vi "macro_FlyWheel_Sim_Execute.vi"() -> ()   [LabVIEW 2019, in "Trajectory_Library.lvlib"]
uses:
  Trajectory_Library.lvlib
  Enum/DCMOTOR_TYPES_ENUM.ctl
  BatterySim_CalculateLoadedBatteryVoltage.vi
panel:
  in  "Motor Dmd (CO)":dbl
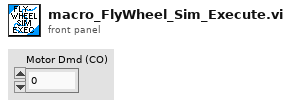
[diagram p1: front panel]
types:
  T1 = typedef "Trajectory_Library.lvlib/DCMOTOR_TYPES_ENUM.ctl" = enum16{"CIM", "AndyMark 9015", "Andy Mark RS 775 125", "Bag", "BaneBots RS 550", "BaneBots RS 775", "Falcon 500", "Mini CIM", "NEO", "NEO 550", "Romi BuiltIn", "Vex 775 Pro", "Snow Blower AM 2235A", "Bosch Seat AM 3493"}
  T2 = typedef "Trajectory_Library.lvlib/FLYWHEEL_SIM_MODEL_PARAMS.ctl" = cluster{"DCMOTOR_TYPES":T1, "Num Motors":i32, "Gearing":dbl, "MOI kgm2":dbl, "Meas Std Dev":dbl}
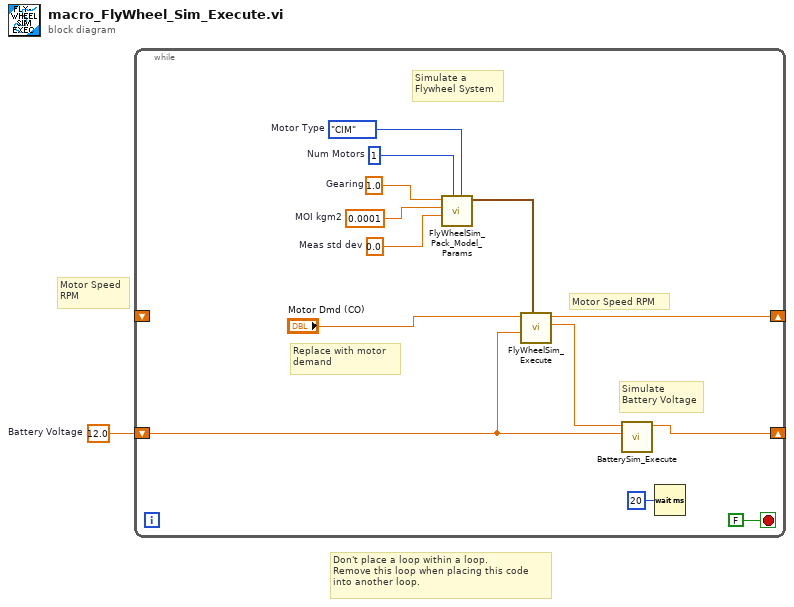
[diagram p0: block diagram]
diagram:
  w1 = 12.0  # Battery Voltage
  # "Don't place a loop within a loop. \nRemove this loop when placing this code\ninto another loop."
  # "Motor Speed\nRPM"
  n1 = while {
    shift-right: [w5] -> _
    shift-left: w1 -> [w2]
    shift-right: [w3] -> _
    shift-left: _ -> [_]
    stop <- FALSE stop-if-true
    w9 = 1.0  # Gearing
    w10 = 0.0001  # MOI kgm2
    w11 = 0.0  # Meas std dev
    w13 = 1  # Num Motors
    w14 = DCMOTOR_TYPES_ENUM."CIM"  # Motor Type
    # "Motor Speed RPM"
    # "Replace with motor \ndemand"
    # "Simulate\nBattery Voltage"
    # "Simulate a \nFlywheel System"
    n2 = call "FlyWheelSim_Pack_Model_Params.vi"("DCMOTOR_TYPES"=w14, "Num Motors"=w13, "Meas Std Dev"=w11, "MOI kgm2"=w10, "Gearing"=w9) -> ("FlyWheelSim_Model _Params"=w12:T2)  [unwired: 6 in]
    n3 = call "FlyWheelSim_Execute.vi"("FlyWheelSim_Model _Params"=w12, "Battery Volts"=w2, "Motor Dmd"="Motor Dmd (CO)") -> ("Motor Current"=w6:dbl, "Velocity_RPM"=w3:dbl)  [unwired: 5 in, 2 out]
    n4 = call "BatterySim_Execute.vi"("Nominal Battery Voltage"=w2, "Current"=w6) -> ("Voltage"=w5:dbl)  [unwired: 9 in]
    n5 = Wait (ms)(milliseconds to wait=u32 20) -> ()  [unwired: 1 out]
  }
